vi "CAL_PRESSURE_TRANSDUCER 2016.vi"(7 "Array in":refnum<k24>[](array[refnum]), 8 "error in (no error)":errorcluster, 9 "Descriptions":string[](array[string]), 10 "Sensor Cluster":T1, 11 "pressure_slope_IN":dbl=51.35 format="%.2f") -> (0 "error out":errorcluster, 2 "Sensor Cluster 2":T1, 3 "pressure_slope_OUT":dbl=51.35 format="%.2f", 5 "Array out":refnum<k24>[](array[refnum]))   [LabVIEW 2016]
uses:
  Waterloo DAQ/controls/MCC DAQ Readings.ctl
  C:/Program Files (x86)/National Instruments/LabVIEW 2016/vi.lib/ULx/ULx_LV.dll
  KPRO_lv2015/ad interface/Global_SIM_switch.vi
  KPRO_lv2015/Kpro Globals.vi
panel:
  out "ok":bool
  out "zero":bool
  out "Pressure":dbl format="%.2f"
  in  "ok":bool
  in  "zero":bool
  # "PRESSURE TRANSDUCER CALIBRATION"
  # "(step 1)"
  # "Fill graduated cylinder to 750 mL water.\nSubmerge Kpro effluent and start flow.\nStop flow at 800 mL of water (1 foot).\nAllow pressure to equilibrate and press zero."
  # "(step 2)"
  # "Hold Kpro effluent facing up and 5' above the floor.\nTurn Kpro flow on briefly to fill the Kpro line.\nTurn Kpro flow off again.\nPress OK when pressure has equilibrated"
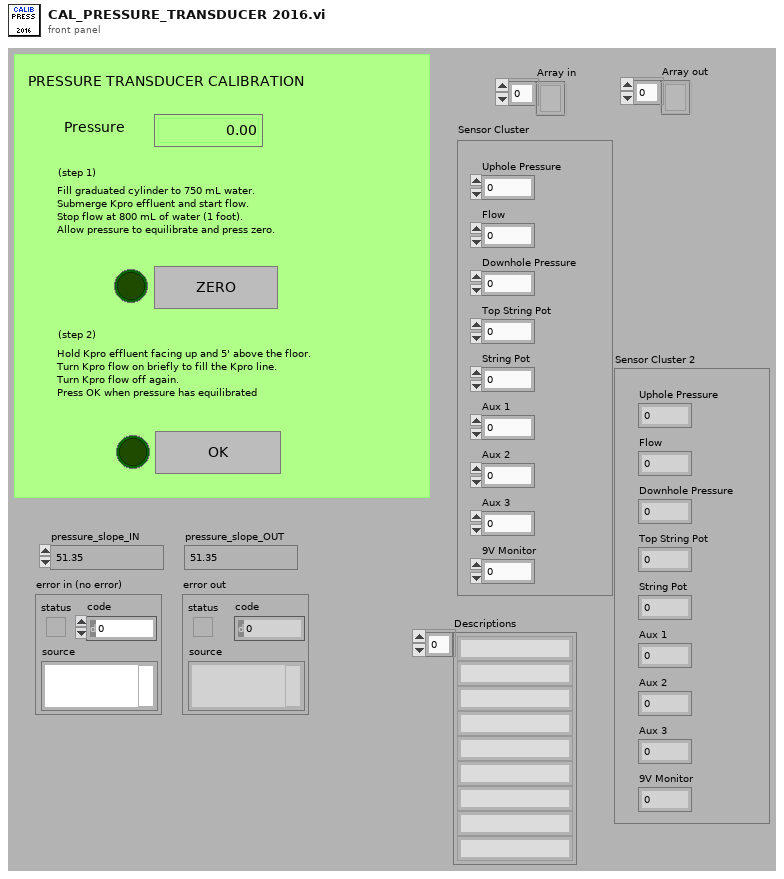
[diagram p1: front panel]
types:
  T1 = typedef "MCC DAQ Readings.ctl" = cluster{"Uphole Pressure":dbl, "Flow":dbl, "Downhole Pressure":dbl, "Top String Pot":dbl, "String Pot":dbl, "Aux 1":dbl, "Aux 2":dbl, "Aux 3":dbl, "9V Monitor":dbl}
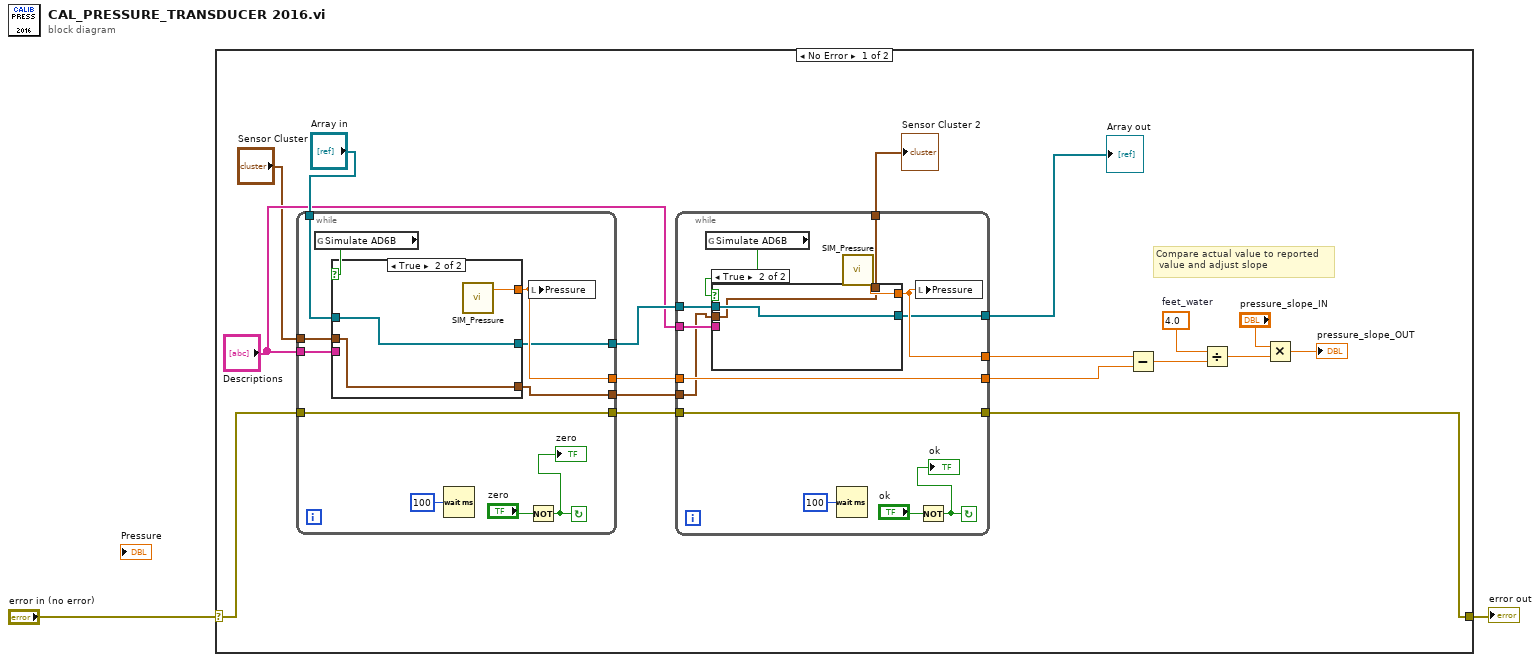
[diagram p0: block diagram]
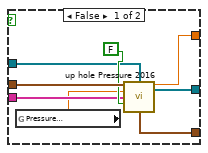
[diagram p2: hidden frame]
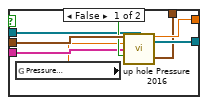
[diagram p3: hidden frame]
diagram:
  n1 = case shown="No Error" "error in (no error)" {
    selector: "error in (no error)" -> [w20 w66]
    tunnel: [w18 w66] -> w2
    frame No Error {
      w16 = 4.0  # feet_water
      # "Compare actual value to reported\n value and adjust slope"
      n2 = while {
        tunnel: [w28] -> w10
        tunnel: [w30] -> w19
        tunnel: w20 -> [w30]
        tunnel: "Sensor Cluster" -> [w25]
        tunnel: "Array in" -> [w24]
        tunnel: [w23] -> w8
        tunnel: "Descriptions" -> [w22]
        tunnel: [w21] -> w4
        stop <- w26 continue-if-true
        n3 = global read "Global_SIM_switch.vi" "Simulate AD6B"() -> (w29:bool)
        n4 = case shown="True" w29 {
          tunnel: [w37 w42] -> w28
          tunnel: w25 -> [w39 w40]
          tunnel: w24 -> [w36 w41]
          tunnel: [w35 w41] -> w23
          tunnel: w22 -> [w34 _]
          tunnel: [w32 w40] -> w21
          frame False {
            n5 = global read "Kpro Globals.vi" "Pressure \nSlope"() -> (w33:dbl)
            n6 = call "up hole Pressure 2016.vi"("Sensor Cluster"=w39, "Array in"=w36, "Pressure \nSlope"=w33, "Descriptions"=w34, "Zero Pressure\n(F = leave as is)"=FALSE ("Zero Pressure\n(F = leave as is)")) -> ("Array out"=w35:refnum<k24>[], "Uphole Pressure"=w37:dbl, "Sensor Cluster 2"=w32:T1)  [unwired: 8 in]
          }
          frame True {
            n7 = call "SIM_Pressure.vi"() -> ("Pressure"=w42:dbl)  [unwired: 11 in]
          }
        }
        n8 = Wait (ms)(milliseconds to wait=u32 100) -> ()  [unwired: 1 out]
        n9 = Not(x="zero") -> (.not. x?=w26:bool)
        "zero" <- w26
        n10 = local write "Pressure"(w28) -> ()
      }
      n11 = while {
        tunnel: w10 -> [w52]
        tunnel: [w49] -> w13
        tunnel: [w52] -> w17
        tunnel: w19 -> [w53]
        tunnel: [w53] -> w18
        tunnel: w8 -> [w47]
        tunnel: [w46] -> w7
        tunnel: "Descriptions" -> [w45]
        tunnel: w4 -> [w44]
        tunnel: [w43] -> w3
        stop <- w50 continue-if-true
        n12 = global read "Global_SIM_switch.vi" "Simulate AD6B"() -> (w48:bool)
        n13 = case shown="True" w48 {
          tunnel: [w60 w65] -> w49
          tunnel: w44 -> [w62 w63]
          tunnel: w47 -> [w59 w64]
          tunnel: [w58 w64] -> w46
          tunnel: w45 -> [w57 _]
          tunnel: [w55 w63] -> w43
          frame False {
            n14 = global read "Kpro Globals.vi" "Pressure \nSlope"() -> (w56:dbl)
            n15 = call "up hole Pressure 2016.vi"("Sensor Cluster"=w62, "Array in"=w59, "Pressure \nSlope"=w56, "Descriptions"=w57, "Zero Pressure\n(F = leave as is)"=FALSE ("Zero Pressure\n(F = leave as is)")) -> ("Array out"=w58:refnum<k24>[], "Uphole Pressure"=w60:dbl, "Sensor Cluster 2"=w55:T1)  [unwired: 8 in]
          }
          frame True {
            n16 = call "SIM_Pressure.vi"() -> ("Pressure"=w65:dbl)  [unwired: 11 in]
          }
        }
        n17 = Wait (ms)(milliseconds to wait=u32 100) -> ()  [unwired: 1 out]
        n18 = local write "Pressure"(w49) -> ()
        n19 = Not(x="ok") -> (.not. x?=w50:bool)
        "ok" <- w50
      }
      "Array out" <- w7
      "Sensor Cluster 2" <- w3
      n20 = Subtract(x=w13, y=w17) -> (x-y=w12:dbl)
      n21 = Divide(x=w16, y=w12) -> (x/y=w11:dbl)
      n22 = Multiply(x="pressure_slope_IN", y=w11) -> (x*y=→"pressure_slope_OUT":dbl)
    }
    frame Error {
    }
  }
  "error out" <- w2
